vi "Parse TimeStamp String.vi"(11 "date/time string":string) -> ()   [LabVIEW 2014]
panel:
  out "Resulting Time Stamp":timestamp
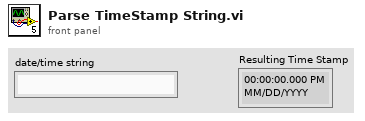
[diagram p1: front panel]
types:
  T1 = cluster{"second":i32, "minute":i32, "hour":i32, "day of month":i32, "month":i32, "year":i32, "day of week":i32, "day of year":i32, "is DST":i32}
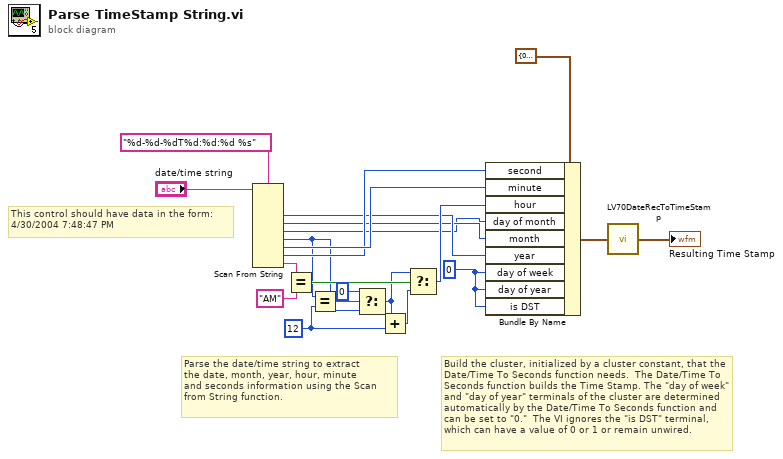
[diagram p0: block diagram]
diagram:
  w8 = 12 ("y")
  w16 = 0
  # "This control should have data in the form:\n4/30/2004 7:48:47 PM"
  # "Build the cluster, initialized by a cluster constant, that the Date/Time To Seconds function needs.  The Date/Time To Seconds function builds the Time Stamp. The \"day of week\" and \"day of year\" terminals of the cluster are determined automatically by the Date/Time To Seconds function and can be set to \"0.\"  The VI ignores the \"is DST\" terminal, which can have a value of 0 or 1 or remain unwired."
  # "Parse the date/time string to extract \nthe date, month, year, hour, minute \nand seconds information using the Scan\nfrom String function."
  n1 = Scan From String "Scan From String"(format string="%d-%d-%dT%d:%d:%d %s", input string="date/time string") -> (output 1=w3:i32, output 2=w2:i32, output 3=w1:i32, output 4=w6:i32, output 5=w15:i32, output 6=w14:i32, output 7=w13:string)  [unwired: 9 in, 3 out]
  n2 = Equal?(x=w13, y="AM") -> (x = y?=w9:bool)
  n3 = Equal?(x=w6, y=w8) -> (x = y?=w7:bool)
  n4 = Select(t=0, s=w7, f=w6) -> (s? t:f=w5:i32)
  n5 = Add(x=w5, y=w8) -> (x+y=w10:i32)
  n6 = Select(t=w5, s=w9, f=w10) -> (s? t:f=w11:i32)
  n7 = Bundle By Name(cluster=T1 {"second"=0, "minute"=0, "hour"=0, "day of month"=0, "month"=0, "year"=0, "day of week"=0, "day of year"=0, "is DST"=0} ("date time rec"), "second"=w14, "minute"=w15, "hour"=w11, "day of month"=w1, "month"=w2, "year"=w3, "day of week"=w16, "day of year"=w16, "is DST"=w16) -> (w17:T1)
  n8 = call <vilib>:"LV70DateRecToTimeStamp.vi"("date time rec"=w17) -> ("Time Stamp"=→"Resulting Time Stamp":timestamp)
